vi "拖曳动作.vi"() -> ()   [LabVIEW 2014]
panel:
  in  "Boolean":bool
  in  "列表框":i32(listbox)
  in  "列表框":i32(listbox)
  # "Drag"
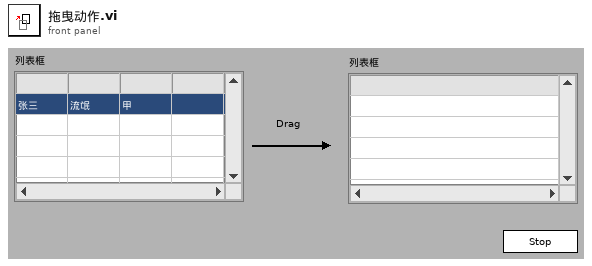
[diagram p1: front panel]
types:
  T1 = cluster{"data name":string, "drag data":variant}[]
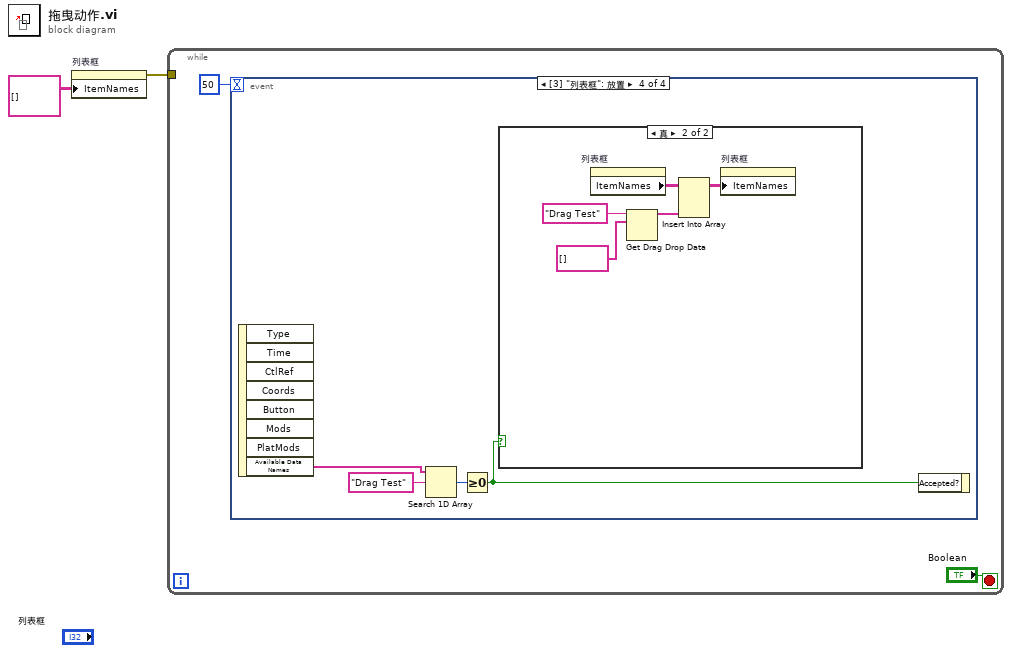
[diagram p0: block diagram]
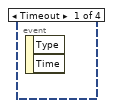
[diagram p2: hidden frame]
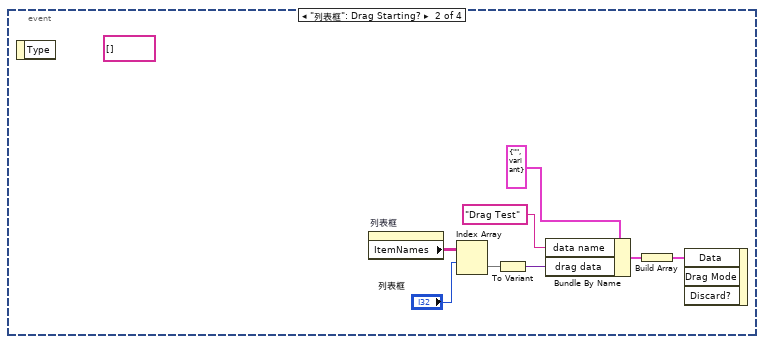
[diagram p3: hidden frame]
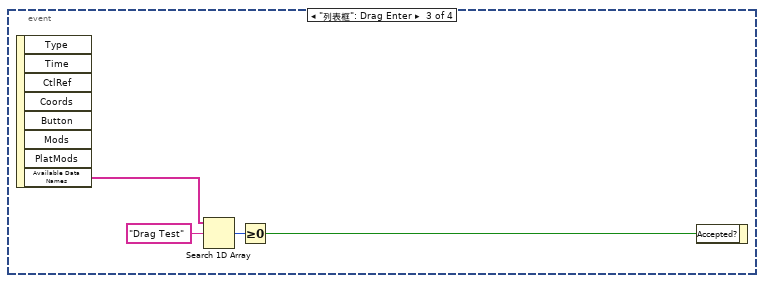
[diagram p4: hidden frame]
diagram:
  n1 = property on="列表框" class="MCListbox (严格)"("ItemNames"=string[][] [] ("Item Names")) -> (error out=w2:errorcluster)  [unwired: 2 in, 1 out]
  n2 = while {
    tunnel: w2 -> [_]
    stop <- "Boolean" stop-if-true
    n3 = event shown="[3] \"列表框\": 放置" {
      selector: _ -> [_ _ _ _]
      dyn-events: _ -> [_ _ _ _]
      timeout: 50 -> [_ _ _ _]
      event Timeout {
        n4 = event-data() -> ()  [unwired: 3 out]
      }
      event "列表框": Drag Starting? {
        (unwired) string[] [] ("subarray")
        n5 = event-data() -> ()  [unwired: 2 out]
        n6 = property on="列表框" class="MCListbox (严格)"() -> ("ItemNames"=w12:string[][])  [unwired: 2 in, 2 out]
        n7 = Index Array(array=w12, index (row)="列表框") -> (element=w6:string[])  [unwired: 1 in]
        n8 = To Variant(anything=w6) -> (Variant=w5:variant)
        n9 = Bundle By Name(cluster=cluster{"data name":string, "drag data":variant} {"data name"="", "drag data"=variant}, "data name"="Drag Test", "drag data"=w5) -> (w9:cluster{"data name":string, "drag data":variant})
        n10 = Build Array(w9) -> (w8:T1)
        n11 = event-data("Data"=w8) -> ()  [unwired: 1 in, 3 out]
      }
      event "列表框": Drag Enter {
        n12 = event-data() -> ("Available Data Names"=w16:string[])  [unwired: 8 out]
        n13 = Search 1D Array(1D array=w16, element="Drag Test") -> (index of element=w14:i32)  [unwired: 1 out]
        n14 = Greater Or Equal To 0?(x=w14) -> (x >= 0?=w13:bool)
        n15 = event-data("Accepted?"=w13) -> ()  [unwired: 1 in, 1 out]
      }
      event "列表框": Drop {
        n16 = event-data() -> ("Available Data Names"=w18:string[])  [unwired: 8 out]
        n17 = Search 1D Array(1D array=w18, element="Drag Test") -> (index of element=w19:i32)  [unwired: 1 out]
        n18 = Greater Or Equal To 0?(x=w19) -> (x >= 0?=w17:bool)
        n19 = case shown="真" w17 {
          frame False {
          }
          frame True {
            n20 = property on="列表框" class="MCListbox (严格)"() -> ("ItemNames"=w23:string[][])  [unwired: 2 in, 2 out]
            n21 = Get Drag Drop Data(8:string[] [] ("subarray"), 9:"Drag Test" ("data name")) -> (3:w22:string[])  [unwired: 1 in, 1 out]
            n22 = Insert Into Array(array=w23, new element=w22) -> (w21:string[][])  [unwired: 2 in]
            n23 = property on="列表框" class="MCListbox (严格)"("ItemNames"=w21) -> ()  [unwired: 2 in, 2 out]
          }
        }
        n24 = event-data("Accepted?"=w17) -> ()  [unwired: 1 in, 1 out]
      }
    }
  }
